vi "SupportedHardware.vi"() -> (3 "Supported Hardware":string[](array[string]))   [LabVIEW 2015]
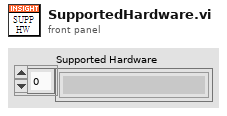
[diagram p1: front panel]
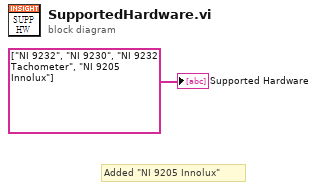
[diagram p0: block diagram]
diagram:
  # "Added \"NI 9205 Innolux\""
  "Supported Hardware" <- string[] ["NI 9232", "NI 9230", "NI 9232 Tachometer", "NI 9205 Innolux"]
